vi "time2access.vi"(1 "time stamp":timestamp) -> (0 "date/time string":string)   [LabVIEW 2010]
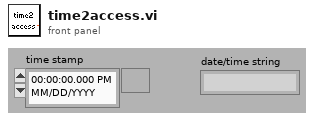
[diagram p1: front panel]
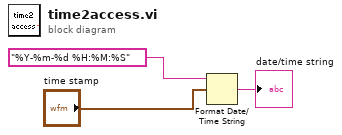
[diagram p0: block diagram]
diagram:
  n1 = Format Date/Time String(time format string (%c)="%Y-%m-%d %H:%M:%S", seconds (now)="time stamp") -> (date/time string=→"date/time string":string)  [unwired: 1 in]
